vi "arduinoDetachServo.vi"(0 "channel":u8 max=15 step=1) -> ()   [LabVIEW 2012]
uses:
  GlobalArduino.vi
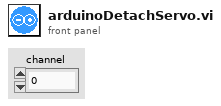
[diagram p1: front panel]
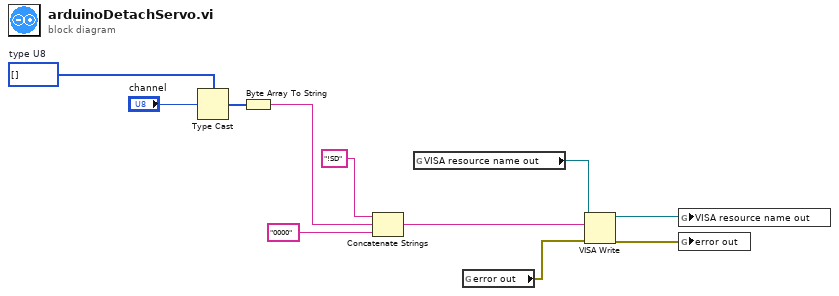
[diagram p0: block diagram]
diagram:
  w2 = u8[] []  # type U8
  n1 = Type Cast(type=w2, x="channel") -> (*(type *) &x=w9:u8[])
  n2 = Byte Array To String(unsigned byte array=w9) -> (string=w10:string)
  n3 = Concatenate Strings("!SD" ("string"), w10, "0000" ("string")) -> (w7:string)
  n4 = global read "GlobalArduino.vi" "VISA resource name out"() -> (w6:refnum<visa-resource-name>)
  n5 = global read "GlobalArduino.vi" "error out"() -> (w4:errorcluster)
  n6 = VISA Write(VISA resource name=w6, write buffer=w7, error in (no error)=w4) -> (VISA resource name out=w5:refnum<visa-resource-name>, error out=w3:errorcluster)  [unwired: 1 out]
  n7 = global write "GlobalArduino.vi" "VISA resource name out"(w5) -> ()
  n8 = global write "GlobalArduino.vi" "error out"(w3) -> ()
